vi "Simple Case Structure Temperature Controller.vi"() -> ()   [LabVIEW 2013]
uses:
  <vilib>/Analysis/baseanly.llb/Mean (DBL).vi
  <vilib>/Analysis/NI_AALBase.lvlib
panel:
  in  "Temperature Control":dbl(slide) scale=0.0..2500.0
  out "Heating Boolean":bool
  out "Mean":dbl format="%0.2f"
  out "Current Mean":dbl
  out "Current Temperature":dbl
  out "Min value":dbl
  out "Max value":dbl
  in  "Stop Button":bool
  out "History":dbl(graph)
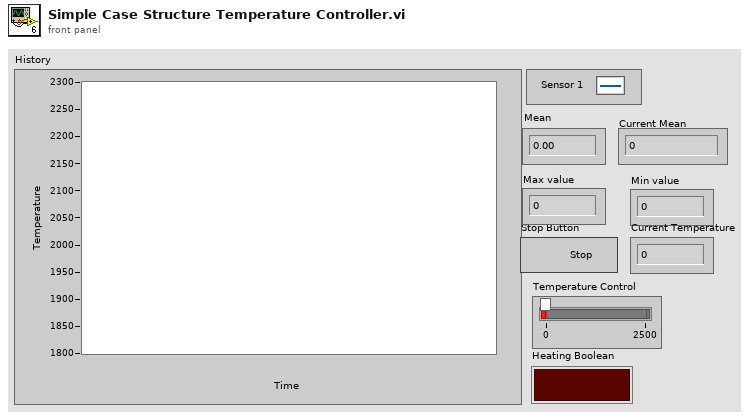
[diagram p1: front panel]
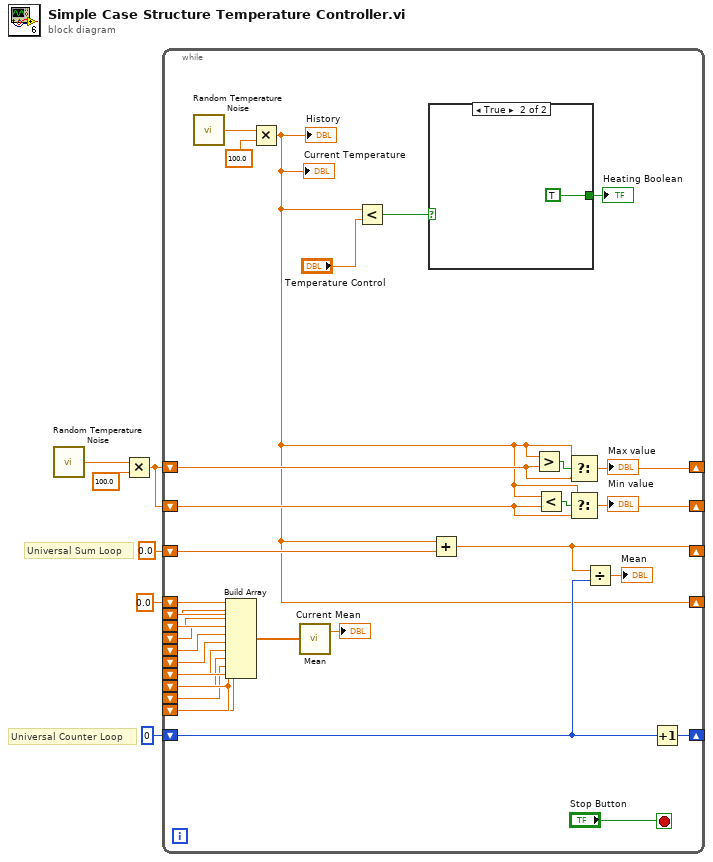
[diagram p0: block diagram]
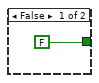
[diagram p2: hidden frame]
diagram:
  w1 = 0.0
  # "Universal Sum Loop"
  # "Universal Counter Loop"
  n1 = call "Random Temperature Noise.vi"() -> ("Temperature"=w5:dbl)  [unwired: 1 in]
  n2 = Multiply(x=w5, y=100.0) -> (x*y=w3:dbl)
  n3 = while {
    shift-right: [w15] -> _
    shift-left: 0.0 -> [w14]
    shift-right: [w31] -> _
    shift-left: w3 -> [w29]
    shift-right: [w30] -> _
    shift-left: w3 -> [w28]
    shift-right: [w10] -> _
    shift-left: w1 -> [w25]
    shift-left: w1 -> [w24]
    shift-left: w1 -> [w16]
    shift-left: w1 -> [w23]
    shift-left: w1 -> [w18]
    shift-left: w1 -> [w19]
    shift-right: [w26] -> _
    shift-left: 0 -> [w12]
    shift-left: w1 -> [w17]
    shift-left: w1 -> [w22]
    shift-left: w1 -> [w20]
    shift-left: w1 -> [w21]
    stop <- "Stop Button" stop-if-true
    n4 = call "Random Temperature Noise.vi"() -> ("Temperature"=w34:dbl)  [unwired: 1 in]
    n5 = Build Array(w25, w24, w23, w22, w21, w20, w19, w18, w17, w16) -> (w7:dbl[])
    n6 = Multiply(x=w34, y=100.0) -> (x*y=w10:dbl)
    "History" <- w10
    "Current Temperature" <- w10
    n7 = call-poly <vilib>:"Mean.vi"("X"=w7) -> ("mean"=→"Current Mean":dbl)  [unwired: 1 out]
    n8 = Less?(x=w10, y="Temperature Control") -> (x < y?=w11:bool)
    n9 = case shown="True" w11 {
      tunnel: [FALSE TRUE] -> w8
      frame False {
      }
      frame True {
      }
    }
    "Heating Boolean" <- w8
    n10 = Add(x=w10, y=w14) -> (x+y=w15:dbl)
    n11 = Greater?(x=w10, y=w29) -> (0:w33:bool)
    n12 = Less?(x=w10, y=w28) -> (x < y?=w32:bool)
    n13 = Select(t=w10, s=w33, f=w29) -> (s? t:f=w31:dbl)
    "Max value" <- w31
    n14 = Select(t=w10, s=w32, f=w28) -> (s? t:f=w30:dbl)
    "Min value" <- w30
    n15 = Divide(x=w15, y=w12) -> (x/y=→"Mean":dbl)
    n16 = Increment(x=w12) -> (x+1=w26:i32)
  }
